vi "Write A.vi"(8 "error in (no error)":errorcluster, 10 "A":dbl, 11 "Add in":refnum<class "Add.lvclass">) -> (0 "error out":errorcluster, 3 "Add out":refnum<class "Add.lvclass">)   [LabVIEW 2023, in "Add.lvclass"]
uses:
  Add.lvclass
  Add.lvclass/Add.ctl
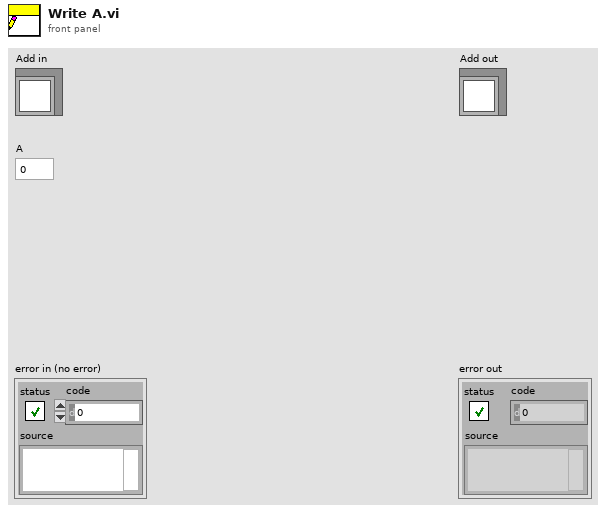
[diagram p1: front panel]
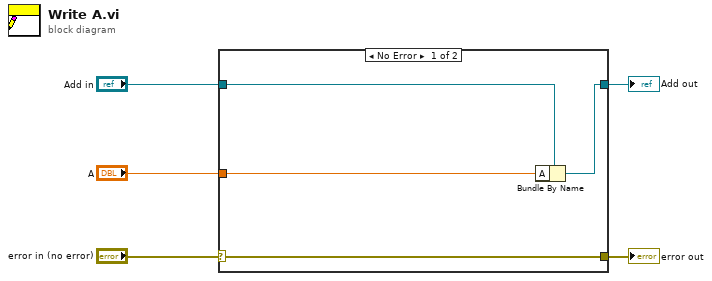
[diagram p0: block diagram]
diagram:
  n1 = case shown="No Error" "error in (no error)" {
    selector: "error in (no error)" -> [w9 w10]
    tunnel: [w9 w10] -> w4
    tunnel: [w7 w11] -> w2
    tunnel: "Add in" -> [w8 w11]
    tunnel: "A" -> [w6 _]
    frame No Error {
      n2 = Bundle By Name(cluster=w8, "A"=w6) -> (w7:refnum<class "Add.lvclass">)
    }
    frame Error {
    }
  }
  "error out" <- w4
  "Add out" <- w2
